vi "AE Group SR Data (SubVI).vi"(5 "Year":i16, 7 "Week":i16, 8 "error in (no error)":errorcluster, 10 "AE-Group":string, 11 "Report DVR in":refnum<data-value>) -> (0 "error out":errorcluster, 2 "Stats Out":T1)   [LabVIEW 2018, in "DS_Lib.lvlib" / "SRReportParser.lvlib"]
uses:
  SRReportParser.lvlib
  TypeDefs/Weekly_SR_Stats.ctl
  Modules/Private Controls/Report Data Cluster.ctl
  Modules/Private Controls/Data Raw.ctl
  Modules/Data Operations.lvlib
panel:
  out "Report DVR out":refnum<data-value>
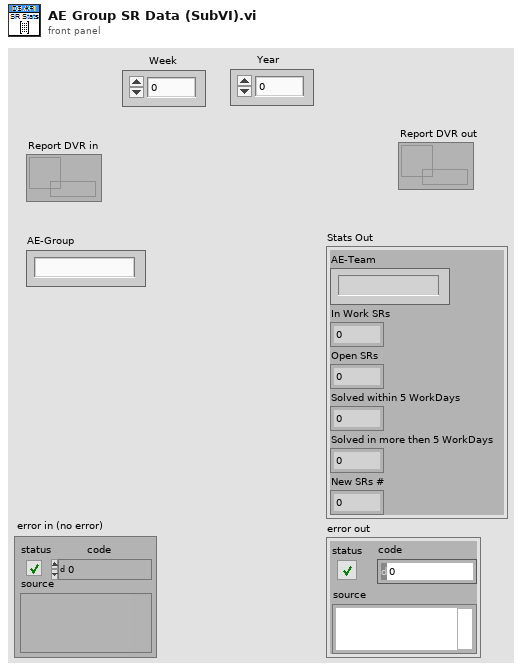
[diagram p1: front panel]
types:
  T1 = typedef "DS_Lib.lvlib/SRReportParser.lvlib/Weekly_SR_Stats.ctl" = cluster{"AE-Team":string, "In Work SRs":i32, "Open SRs":i32, "Solved within 5 WorkDays":i32, "Solved in more then 5 WorkDays":i32, "New SRs #":i32}
  T2 = typedef "Data Operations.lvlib/Report Data Cluster.ctl" = cluster{"Headers":cluster{"Start Date":timestamp, "End Date":timestamp, "SR Status String":string[], "AE Owner String":string[]}, "Data":T3[]}
  T3 = typedef "Data Operations.lvlib/Data Raw.ctl" = cluster{"SR Number":string, "Status":string, "Summary":string, "AE Owner":string, "AE Group":string, "Contact":string, "SurveyData":cluster{"Resolution Time":dbl, "Total Satisfaction":dbl, "Response Time":dbl, "Courtesy":dbl, "Problem Solved":dbl, "Level of effort":dbl}, "Time Data":cluster{"Last Update Date":timestamp, "Creation Date":timestamp, "Creation week":i16, "Last Update Week":i16, "Creation Year":i16}}
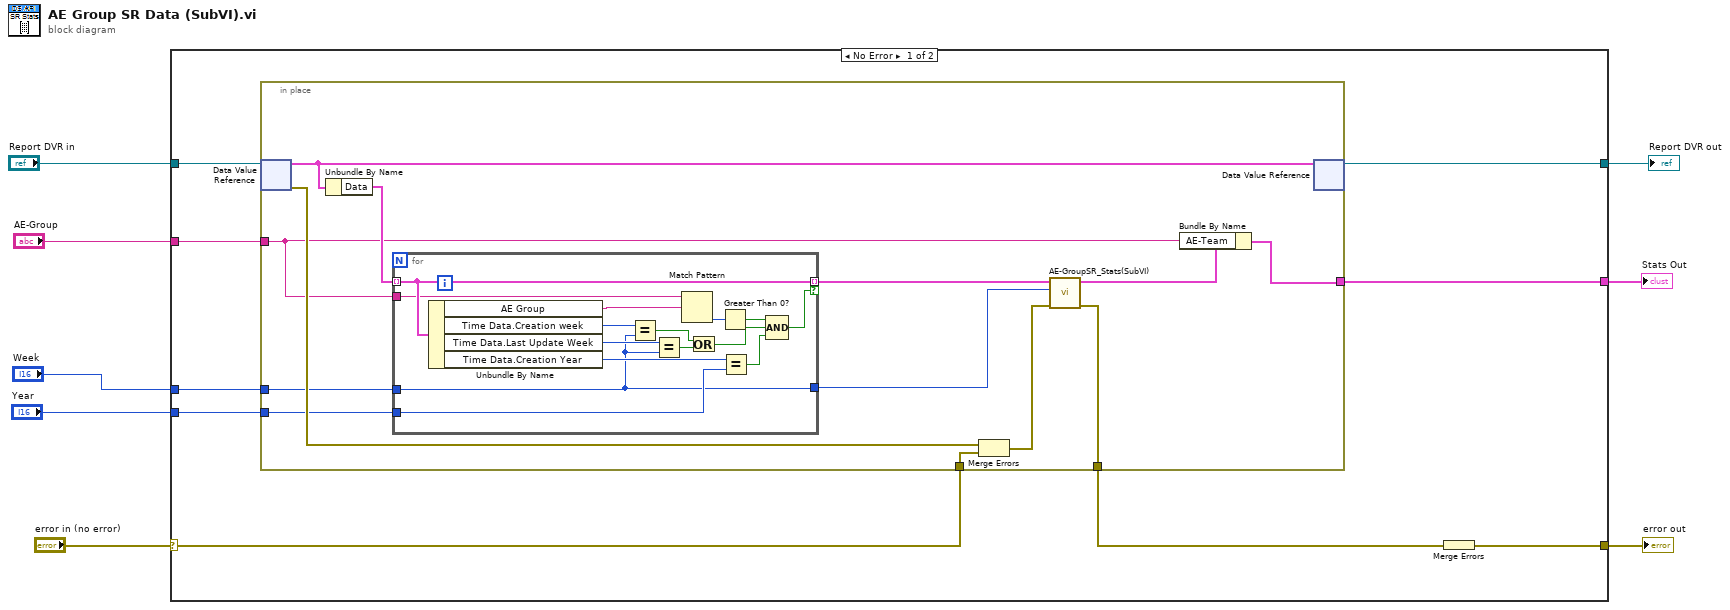
[diagram p0: block diagram]
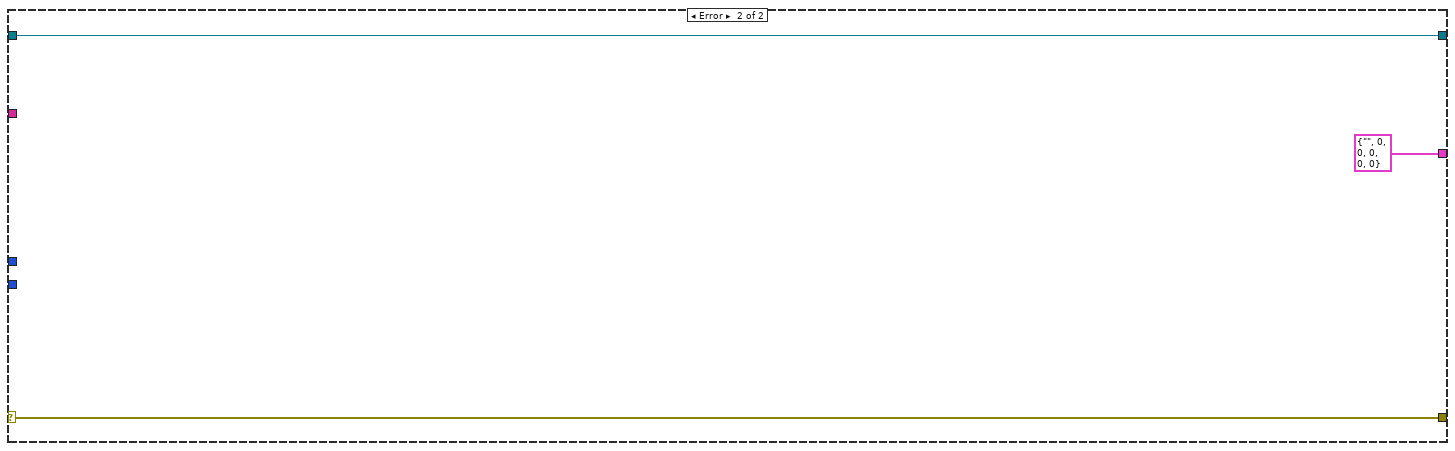
[diagram p2: hidden frame]
diagram:
  n1 = case shown="No Error" "error in (no error)" {
    selector: "error in (no error)" -> [w12 w48]
    tunnel: [w16 w48] -> w8
    tunnel: "Report DVR in" -> [w17 w46]
    tunnel: "Week" -> [w15 _]
    tunnel: "AE-Group" -> [w14 _]
    tunnel: [w13 T1 {"AE-Team"="", "In Work SRs"=0, "Open SRs"=0, "Solved within 5 WorkDays"=0, "Solved in more then 5 WorkDays"=0, "New SRs #"=0} ("Stats Out")] -> w4
    tunnel: [w10 w46] -> w2
    tunnel: "Year" -> [w9 _]
    frame No Error {
      n2 = in-place {
        in-place-border: w15 -> [w24]
        in-place-border: w14 -> [w22]
        in-place-border: [w21] -> w13
        in-place-border: w12 -> [w30]
        in-place-border: [w26] -> w11
        in-place-border: w9 -> [w19]
        n3 = in-place-dvr #1(w17) -> (w20:T2, w29:errorcluster)
        n4 = Unbundle By Name(w20) -> ("Data"=w28:T3[])
        n5 = for {
          tunnel: w28 -> [w45] mode=indexing
          tunnel: w24 -> [w31]
          tunnel: [w45] -> w25 mode=indexing if=w32
          tunnel: w22 -> [w42]
          tunnel: w19 -> [w40]
          tunnel: [w31] -> w18
          n6 = Unbundle By Name(w45) -> ("AE Group"=w44:string, "Time Data.Creation week"=w38:i16, "Time Data.Last Update Week"=w37:i16, "Time Data.Creation Year"=w41:i16)
          n7 = Equal?(x=w38, y=w31) -> (x = y?=w35:bool)
          n8 = Equal?(x=w37, y=w31) -> (x = y?=w36:bool)
          n9 = Match Pattern(string=w42, regular expression=w44) -> (offset past match=w43:i32)  [unwired: 1 in, 3 out]
          n10 = Or(x=w35, y=w36) -> (x .or. y?=w34:bool)
          n11 = Greater Than 0?(x=w43) -> (x > 0?=w39:bool)
          n12 = Equal?(x=w41, y=w40) -> (x = y?=w33:bool)
          n13 = Compound Arithmetic op=AND(w39, w34, w33) -> (w32:bool)
        }
        n14 = Merge Errors(w29, w30) -> (w27:errorcluster)
        n15 = call "AE-GroupSR_Stats(SubVI).vi"("error in (no error)"=w27, "Search Week"=w18, "Report Data"=w25) -> ("error out"=w26:errorcluster, "Stats Out"=w23:T1)  [unwired: 7 in]
        n16 = Bundle By Name(cluster=w23, "AE-Team"=w22) -> (w21:T1)
        n17 = in-place-dvr #1(w20) -> (w10:refnum<data-value>)  [unwired: 1 out]
      }
      n18 = Merge Errors(w11) -> (w16:errorcluster)
    }
    frame Error {
    }
  }
  "error out" <- w8
  "Stats Out" <- w4
  "Report DVR out" <- w2
